vi "Construct LVQueue Sink.vi"(6 "Error Action":T1=enum."Ignore Error and Close Sink", 7 "User Shutdown? (F)":bool, 9 "Log Filter":refnum<class "ILogFilter.lvclass">, 10 "LogLevel":T2, 11 "Max Queue size (-1, unlimited)":i32=-1) -> (0 "error out":errorcluster, 3 "LVQueue Sink out":refnum<class "LVQueue Sink.lvclass">)   [LabVIEW 2020, in "MVA Framework.lvlib" / "LVQueue Sink.lvclass"]
uses:
  LVQueue Sink.lvclass
  Composed Log/Types/Log Level.ctl
  Composed Log/Log Sink/Sink Error Actions ENUM.ctl
  Composed Log/ILogFilter/ILogFilter.lvclass
  Composed Log/Types/Log Packet.ctl
  LVQueue Sink.lvclass/LVQueue Sink.ctl
  Composed Log/Log Sink/Log Sink.lvclass/Log Sink.ctl
  Composed Log/Composed Log.lvlib
  Composed Log/Log Sink/Log Sink.lvclass
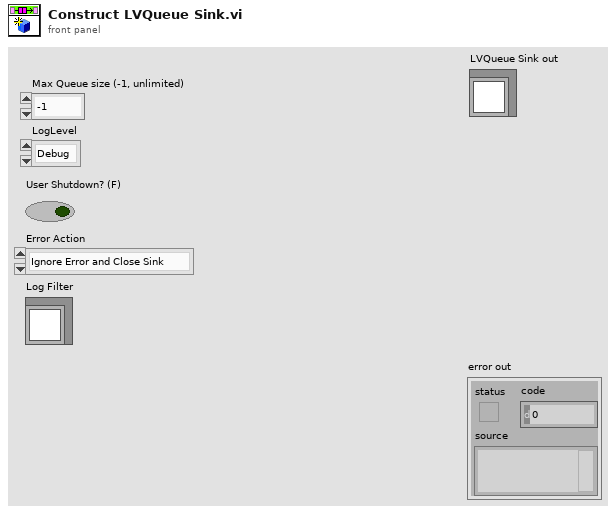
[diagram p1: front panel]
types:
  T1 = typedef "MVA Framework.lvlib/Composed Log.lvlib/Log Sink.lvclass/Sink Error Actions ENUM.ctl" = enum16{"Ignore Error and Continue", "Ignore Error and Close Sink", "Report Error and Close Sink"}
  T2 = typedef "MVA Framework.lvlib/Composed Log.lvlib/Log Level.ctl" = enum16{"Debug", "Info", "Warning", "Error", "Critical"}
  T3 = typedef "MVA Framework.lvlib/Composed Log.lvlib/Log Packet.ctl" = cluster{"Data To Log":string, "Source":string, "Event Level":T2, "Event Time":timestamp}
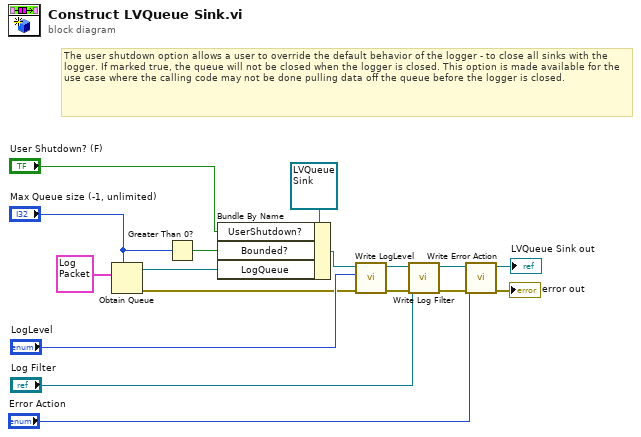
[diagram p0: block diagram]
diagram:
  # "The user shutdown option allows a user to override the default behavior of the logger - to close all sinks with the logger. If marked true, the queue will not be closed when the logger is closed. This option is made available for the use case where the calling code may not be done pulling data off the queue before the logger is closed."
  n1 = Obtain Queue(max queue size (-1, unlimited)="Max Queue size (-1, unlimited)", element data type=T3 {"Data To Log"="", "Source"="", "Event Level"=enum."Debug", "Event Time"=timestamp(0 s since 1904-01-01)} ("Log Packet")) -> (queue out=w16:refnum<queue>, error out=w10:errorcluster)  [unwired: 3 in, 1 out]
  n2 = Greater Than 0?(x="Max Queue size (-1, unlimited)") -> (x > 0?=w13:bool)
  n3 = Bundle By Name(cluster=refnum<class "LVQueue Sink.lvclass"> refnum ("LVQueue Sink in"), "UserShutdown?"="User Shutdown? (F)", "Bounded?"=w13, "LogQueue"=w16) -> (w12:refnum<class "LVQueue Sink.lvclass">)
  n4 = call "Write LogLevel.vi"("error in (no error)"=w10, "LogLevel"="LogLevel", "Log Sink in"=w12) -> ("error out"=w7:errorcluster, "Log Sink in"=w8:refnum<class "LVQueue Sink.lvclass">)  [unwired: 7 in]
  n5 = call "Write Log Filter.vi"("error in (no error)"=w7, "Log Filter"="Log Filter", "Log Sink in"=w8) -> ("error out"=w2:errorcluster, "Log Sink in"=w6:refnum<class "LVQueue Sink.lvclass">)  [unwired: 7 in]
  n6 = call "Write Error Action.vi"("error in (no error)"=w2, "Error Action"="Error Action", "Log Sink in"=w6) -> ("error out"=→"error out":errorcluster, "Log Sink in"=→"LVQueue Sink out":refnum<class "LVQueue Sink.lvclass">)  [unwired: 7 in]
